vi "SwapInstanceVIUnusedName2 60.vi"(6 "Bindata & descr in":T1, 7 "type":i8, 8 "error in (no error)":errorcluster, 9 "dims":u8=3 min=1 max=3, 11 "kwarg_name":string="testarg") -> (0 "error out":errorcluster, 1 "Array 3D":i8[][][](array[numeric]), 2 "Array 2D":i8[][](array[numeric]), 3 "Array 1D":i8[](array[numeric]), 4 "Bindata & descr out":T1, 5 "bindata":u8[](array[numeric]))   [LabVIEW 2018]
uses:
  Bindata&description.ctl
  Bindata description.ctl
  6956e7a2-ec88-45ad-b43c-1ae0634bf051.vi
  c466d00e-71e5-4b21-ada6-455d5c0b5724.vi
  09ea6b2e-535e-4fd6-b41b-9e4a603228e5.vi
  4e2fe0f7-34df-40a0-ad06-71a71370a469.vi
  c466d00e-71e5-4b21-ada6-455d5c0b5724.vi/8f2bb363-1e9a-4340-ac91-adf4b3017f89.vi
  09ea6b2e-535e-4fd6-b41b-9e4a603228e5.vi/c496b00a-17c9-4ce4-b24e-860ce7636337.vi
  4e2fe0f7-34df-40a0-ad06-71a71370a469.vi/ac7f3bf2-bf33-43de-ab43-63b42607039c.vi
  c466d00e-71e5-4b21-ada6-455d5c0b5724.vi/8f2bb363-1e9a-4340-ac91-adf4b3017f89.vi/711ffea0-864c-441c-b6c2-36be3c638376.vi
  09ea6b2e-535e-4fd6-b41b-9e4a603228e5.vi/c496b00a-17c9-4ce4-b24e-860ce7636337.vi/9ee27b7a-e1ba-4bae-a0ac-08bdc29a4a72.vi
  4e2fe0f7-34df-40a0-ad06-71a71370a469.vi/ac7f3bf2-bf33-43de-ab43-63b42607039c.vi/effe006d-959f-46e4-8300-3619c61503da.vi
  c466d00e-71e5-4b21-ada6-455d5c0b5724.vi/8f2bb363-1e9a-4340-ac91-adf4b3017f89.vi/711ffea0-864c-441c-b6c2-36be3c638376.vi/650967db-e859-45a5-8e91-ab66a5541fc5.vi
  09ea6b2e-535e-4fd6-b41b-9e4a603228e5.vi/c496b00a-17c9-4ce4-b24e-860ce7636337.vi/9ee27b7a-e1ba-4bae-a0ac-08bdc29a4a72.vi/1b3912b6-c82f-4139-b79e-636cfde2725c.vi
  4e2fe0f7-34df-40a0-ad06-71a71370a469.vi/ac7f3bf2-bf33-43de-ab43-63b42607039c.vi/effe006d-959f-46e4-8300-3619c61503da.vi/10e633ac-6830-4de4-b20c-5ac8711e5b05.vi
  check ID validity.vi
  LV-Julia_ZMQ-Roundtrip_lib.lvlib
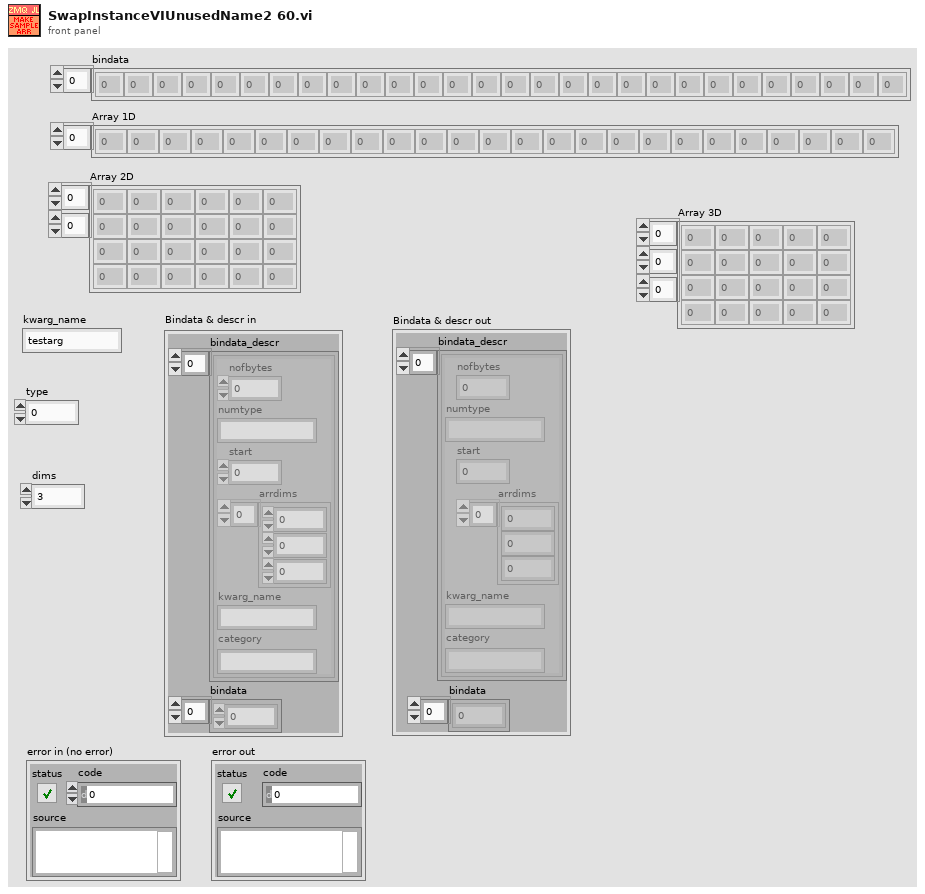
[diagram p1: front panel]
types:
  T1 = typedef "Bindata&description.ctl" = cluster{"bindata_descr":T2[], "bindata":u8[]}
  T2 = typedef "LV-Julia_ZMQ-Roundtrip_lib.lvlib/Bindata description.ctl" = cluster{"nofbytes":i32, "numtype":string, "start":i32, "arrdims":i32[], "kwarg_name":string, "category":string}
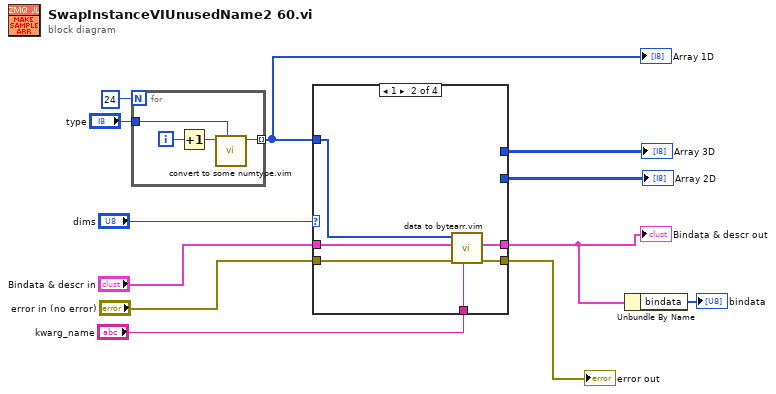
[diagram p0: block diagram]
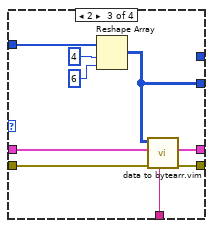
[diagram p3: hidden frame]
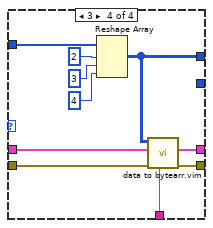
[diagram p4: hidden frame]
diagram:
  n1 = for {
    N: 24 -> [_]
    tunnel: [w14] -> w11 mode=indexing
    tunnel: "type" -> [w13]
    i -> [w16]
    n2 = Increment(x=w16) -> (x+1=w15:i32)
    n3 = call "convert to some numtype.vim"("type"=w13, "Numeric in"=w15) -> ("Numeric out"=w14:i8)  [unwired: 9 in]
  }
  "Array 1D" <- w11
  n4 = case shown="1" "dims" {
    tunnel: [_ _ _ w42] -> w12
    tunnel: w11 -> [_ w23 w30 w38]
    tunnel: "kwarg_name" -> [_ w22 w29 w37]
    tunnel: "error in (no error)" -> [w17 w21 w28 w36]
    tunnel: [w17 w20 w27 w35] -> w5
    tunnel: [_ w19 w26 w34] -> w2
    tunnel: [_ _ w25 _] -> w4
    tunnel: "Bindata & descr in" -> [_ w18 w24 w33]
    frame 0, Default {
    }
    frame 1 {
      n5 = call "data to bytearr.vim"("kwarg_name"=w22, "error in (no error)"=w21, "Bindata & descr in"=w18, "data in"=w23) -> ("error out"=w20:errorcluster, "Bindata & descr out"=w19:T1)  [unwired: 5 in, 1 out]
    }
    frame 2 {
      n6 = Reshape Array(w30, 4 ("dimension size"), 6 ("dimension size")) -> (w25:i8[][])
      n7 = call "data to bytearr.vim"("kwarg_name"=w29, "error in (no error)"=w28, "Bindata & descr in"=w24, "data in"=w25) -> ("error out"=w27:errorcluster, "Bindata & descr out"=w26:T1)  [unwired: 5 in, 1 out]
    }
    frame 3 {
      n8 = Reshape Array(w38, 2 ("dimension size"), 3 ("dimension size"), 4 ("dimension size")) -> (w42:i8[][][])
      n9 = call "data to bytearr.vim"("kwarg_name"=w37, "error in (no error)"=w36, "Bindata & descr in"=w33, "data in"=w42) -> ("error out"=w35:errorcluster, "Bindata & descr out"=w34:T1)  [unwired: 5 in, 1 out]
    }
  }
  "Array 3D" <- w12
  "Bindata & descr out" <- w2
  "error out" <- w5
  "Array 2D" <- w4
  n10 = Unbundle By Name(w2) -> ("bindata"=→"bindata":u8[])
